vi "TSM SSC Digital Configure Time Set Compare Edge Per-Site Per-Pin.vi"(0 "Digital TSM In":T1, 5 "time set":string caption="Time Set", 7 "Per-Site Per-Pin Compare Strobe (s)":dbl[][](array[numeric]), 11 "error in":errorcluster) -> (4 "Digital TSM Out":T1, 15 "error out":errorcluster)   [LabVIEW 2019]
doc: "Configures the strobe edge time for the specified pins. Use this function to modify time set values after applying a timing sheet with the niDigital Apply Levels and Timing VI, or to create time sets programmatically without the use of timing sheets. This function does not modify the timing sheet file or the timing sheet contents that will be used in future calls to niDigital Apply Levels and Timing; it only affects the values of the current timing context."
uses:
  TSM/TSM SSC Digital.ctl
  <vilib>/NI_TestStand_SemiconductorModule/NI_TestStand_Semiconductor_Module.lvlibp/PinMap/Digital Pattern/PinQueryContext/DigitalPatternPinQueryContext.lvclass
  SSC Digital/SSC Digital.ctl
  f849a686-a01d-4d2f-8234-3cebd32d409b.vi
  Shared SubVIs/Trim Whitespace [Inlined].vi
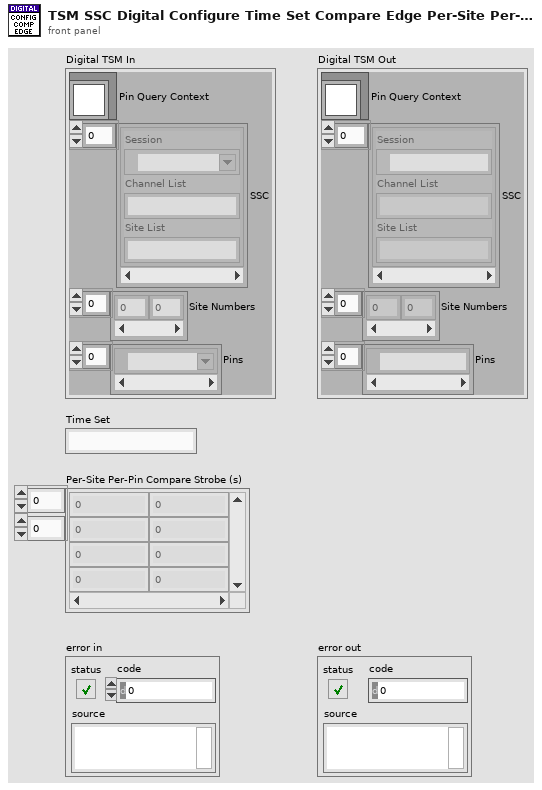
[diagram p1: front panel]
types:
  T1 = typedef "TSM SSC Digital.ctl" = cluster{"Pin Query Context":refnum<class "DigitalPatternPinQueryContext.lvclass">, "SSC":T2[], "Site Numbers":i32[], "Pins":tag[]}
  T2 = typedef "SSC Digital.ctl" = cluster{"Session":refnum<k15>, "Channel List":string, "Site List":string}
  T3 = typedef "Digital 2D Location.ctl" = cluster{"Row":i32, "Col":i32}
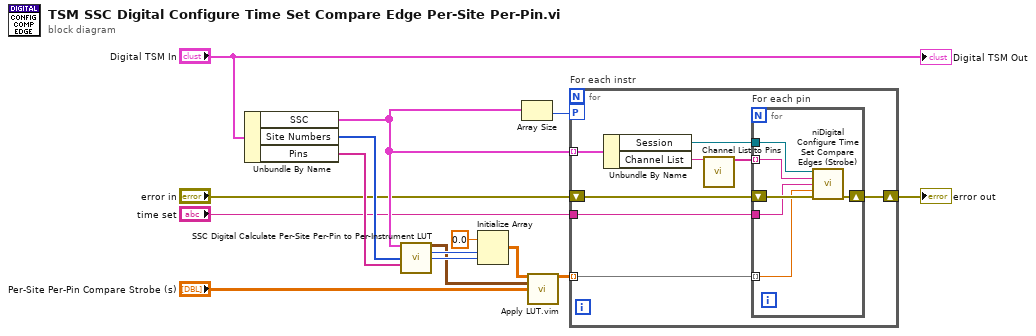
[diagram p0: block diagram]
diagram:
  n1 = Unbundle By Name("Digital TSM In") -> ("SSC"=w6:T2[], "Site Numbers"=w10:i32[], "Pins"=w9:tag[])
  n2 = call "SSC Digital Calculate Per-Site Per-Pin to Per-Instrument LUT.vi"("Digital SSC In"=w6, "Sites"=w10, "Pins"=w9) -> ("Per-Site Per-Pin to Per-Instrument LUT"=w12:T3[][], "Instrument Count"=w15:i32, "Max Sites on Instrument"=w14:i32)  [unwired: 10 in]
  n3 = Initialize Array(0.0 ("element"), w15, w14) -> (w13:dbl[][])
  n4 = Array Size(array=w6) -> (size(s)=w7:i32)
  n5 = call "Apply LUT.vim"("Initialized Array"=w13, "LUT"=w12, "Results to Apply LUT to"="Per-Site Per-Pin Compare Strobe (s)") -> ("Array Out"=w11:dbl[][])  [unwired: 12 in]
  n6 = for "For each instr" {
    tunnel: "time set" -> [w16]
    workers-P: w7 -> [_]
    tunnel: w6 -> [w19] mode=indexing
    tunnel: w11 -> [w21] mode=indexing
    shift-right: [w22] -> w5
    shift-left: "error in" -> [w23]
    n7 = Unbundle By Name(w19) -> ("Session"=w17:refnum<k15>, "Channel List"=w18:string)
    n8 = call "Channel List to Pins.vi"("Channel List"=w18) -> ("Sites and Pins"=w20:string[])  [unwired: 12 in, 2 out]
    n9 = for "For each pin" {
      shift-right: [w28] -> w22
      shift-left: w23 -> [w29]
      tunnel: w20 -> [w26] mode=indexing
      tunnel: w21 -> [w25] mode=indexing
      tunnel: w17 -> [w27]
      tunnel: w16 -> [w24]
      n10 = call <instrlib>:"niDigital Configure Time Set Compare Edges (Strobe).vi"("instrument handle"=w27, "pin list"=w26, "edge set"=w24, "compare strobe (s)"=w25, "error in"=w29) -> ("error out"=w28:errorcluster)  [unwired: 9 in, 1 out]
    }
  }
  "error out" <- w5
  "Digital TSM Out" <- "Digital TSM In"
